vi "calculate_smooth_points.vi"(8 "error in (no error)":errorcluster, 11 "TrajectoryDL120126ArbitraryLine2D in":refnum<class "TrajectoryDL120126ArbitraryLine2D.lvclass">) -> (0 "error out":errorcluster, 2 "number of pixels":i32, 3 "TrajectoryDL120126ArbitraryLine2D out":refnum<class "TrajectoryDL120126ArbitraryLine2D.lvclass">)   [LabVIEW 2010, in "TrajectoryDL120126ArbitraryLine2D.lvclass"]
uses:
  TrajectoryDL120126ArbitraryLine2D.lvclass
  segment_cluster.ctl
  common/classes/SpaceVector/SpaceVector/SpaceVector.lvclass
  TrajectoryDL120126ArbitraryLine2D.lvclass/TrajectoryDL120126ArbitraryLine2D.ctl
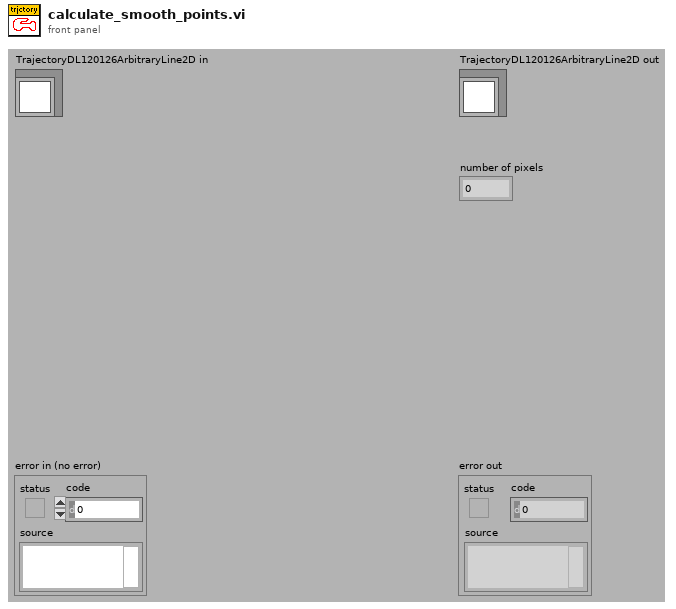
[diagram p1: front panel]
types:
  T1 = typedef "TrajectoryDL120126ArbitraryLine2D.lvclass/segment_cluster.ctl" = cluster{"points":refnum<class "SpaceVector.lvclass">[]}
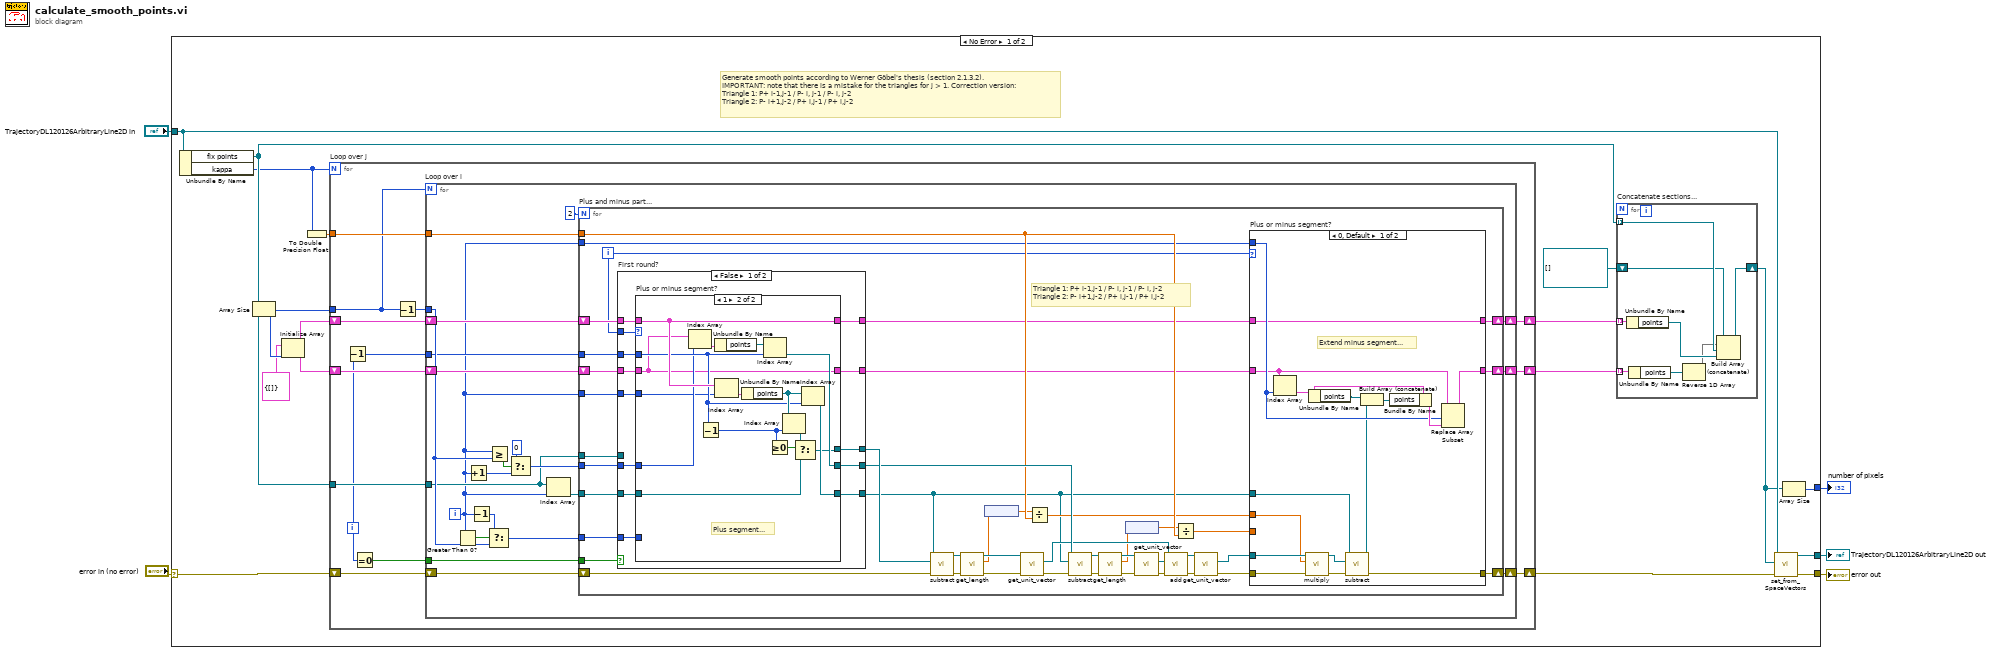
[diagram p0: block diagram]
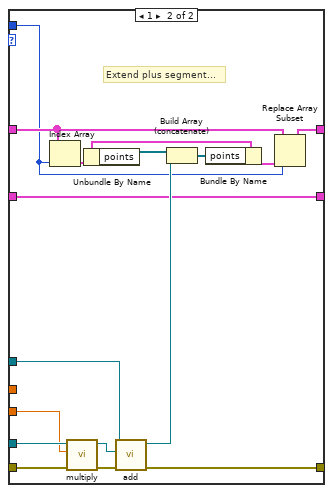
[diagram p2: hidden frame]
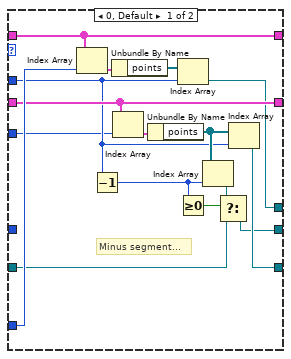
[diagram p3: hidden frame]
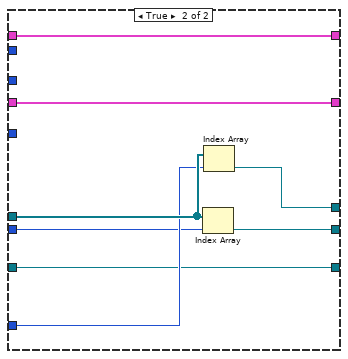
[diagram p4: hidden frame]
diagram:
  n1 = case shown="No Error" "error in (no error)" {
    selector: "error in (no error)" -> [w21 w192]
    tunnel: "TrajectoryDL120126ArbitraryLine2D in" -> [w11 w193]
    tunnel: [w9 w192] -> w3
    tunnel: [w10 w193] -> w2
    tunnel: [w6 _] -> w1
    frame No Error {
      # "Generate smooth points according to Werner Göbel's thesis (section 2.1.3.2). \nIMPORTANT: note that there is a mistake for the triangles for j > 1. Correction version:\nTriangle 1: P+ i-1,j-1 / P- i, j-1 / P- i, j-2\nTriangle 2: P- i+1,j-2 / P+ i,j-1 / P+ i,j-2"
      n2 = Unbundle By Name(w11) -> ("fix points"=w14:refnum<class "SpaceVector.lvclass">[], "kappa"=w13:i32)
      n3 = Array Size(array=w14) -> (size(s)=w18:i32)
      n4 = Initialize Array(T1 {"points"=[]} ("segment"), w18) -> (w16:T1[])
      n5 = To Double Precision Float(number=w13) -> (double precision float=w20:dbl)
      n6 = for "Loop over j" {
        N: w13 -> [_]
        tunnel: w14 -> [w40]
        shift-right: [w41] -> w12
        shift-left: w21 -> [w42]
        shift-right: [w38] -> w19
        shift-left: w16 -> [w39]
        shift-right: [w36] -> w8
        shift-left: w16 -> [w37]
        tunnel: w20 -> [w35]
        tunnel: w18 -> [w31]
        i -> [w33]
        n7 = Decrement(x=w33) -> (x-1=w34:i32)
        n8 = Equal To 0?(x=w33) -> (x = 0?=w32:bool)
        n9 = Decrement(x=w31) -> (x-1=w30:i32)
        n10 = for "Loop over i" {
          N: w31 -> [_]
          shift-right: [w61] -> w41
          shift-left: w42 -> [w63]
          tunnel: w40 -> [w46]
          shift-right: [w59] -> w38
          shift-left: w39 -> [w52]
          shift-right: [w60] -> w36
          shift-left: w37 -> [w50]
          tunnel: w35 -> [w62]
          tunnel: w30 -> [w49]
          tunnel: w34 -> [w47]
          tunnel: w32 -> [w45]
          i -> [w43]
          n11 = Greater Than 0?(x=w43) -> (x > 0?=w58:bool)
          n12 = Increment(x=w43) -> (x+1=w53:i32)
          n13 = Decrement(x=w43) -> (x-1=w57:i32)
          n14 = Select(t=w57, s=w58, f=w49) -> (s? t:f=w51:i32)
          n15 = Greater Or Equal?(x=w43, y=w49) -> (x >= y?=w56:bool)
          n16 = Select(t=0, s=w56, f=w53) -> (s? t:f=w55:i32)
          n17 = Index Array(array=w46, index=w43) -> (element=w48:refnum<class "SpaceVector.lvclass">)
          n18 = for "Plus and minus part..." {
            N: 2 -> [_]
            tunnel: w62 -> [w88]
            tunnel: w55 -> [w77]
            tunnel: w43 -> [w66]
            tunnel: w51 -> [w75]
            tunnel: w48 -> [w73]
            tunnel: w47 -> [w72]
            tunnel: w46 -> [w71]
            tunnel: w45 -> [w70]
            shift-right: [w78] -> w59
            shift-left: w52 -> [w76]
            shift-right: [w79] -> w60
            shift-left: w50 -> [w74]
            shift-right: [w80] -> w61
            shift-left: w63 -> [w104]
            tunnel: w43 -> [w65]
            i -> [w64]
            # "Triangle 1: P+ i-1,j-1 / P- i, j-1 / P- i, j-2\nTriangle 2: P- i+1,j-2 / P+ i,j-1 / P+ i,j-2"
            n19 = case "First round?" shown="False" w70 {
              tunnel: [w144 w187] -> w106
              tunnel: [w146 w188] -> w105
              tunnel: w77 -> [w142 w189]
              tunnel: w76 -> [w148 w185]
              tunnel: w75 -> [w151 w190]
              tunnel: w74 -> [w147 w184]
              tunnel: w73 -> [w150 w186]
              tunnel: w72 -> [w149 _]
              tunnel: w71 -> [_ w191]
              tunnel: [w145 w186] -> w69
              tunnel: [w140 w185] -> w68
              tunnel: [w139 w184] -> w67
              tunnel: w64 -> [w143 _]
              tunnel: w65 -> [w141 _]
              frame False {
                n20 = case "Plus or minus segment?" shown="1" w143 {
                  tunnel: w151 -> [w160 _]
                  tunnel: w150 -> [w159 w175]
                  tunnel: w149 -> [w157 w174]
                  tunnel: w148 -> [w156 w183]
                  tunnel: w147 -> [w158 w168]
                  tunnel: [w153 w173] -> w146
                  tunnel: [w155 w172] -> w145
                  tunnel: [w152 w171] -> w144
                  tunnel: w142 -> [_ w170]
                  tunnel: w141 -> [w154 w169]
                  tunnel: [w156 w183] -> w140
                  tunnel: [w158 w168] -> w139
                  frame 0, Default {
                    # "Minus segment..."
                    n21 = Index Array(array=w156, index=w160) -> (element=w167:T1)
                    n22 = Decrement(x=w157) -> (x-1=w163:i32)
                    n23 = Unbundle By Name(w167) -> ("points"=w166:refnum<class "SpaceVector.lvclass">[])
                    n24 = Index Array(array=w158, index=w154) -> (element=w165:T1)
                    n25 = Unbundle By Name(w165) -> ("points"=w164:refnum<class "SpaceVector.lvclass">[])
                    n26 = Index Array(array=w166, index=w157) -> (element=w152:refnum<class "SpaceVector.lvclass">)
                    n27 = Greater Or Equal To 0?(x=w163) -> (x >= 0?=w162:bool)
                    n28 = Index Array(array=w164, index=w163) -> (element=w161:refnum<class "SpaceVector.lvclass">)
                    n29 = Select(t=w161, s=w162, f=w159) -> (s? t:f=w153:refnum<class "SpaceVector.lvclass">)
                    n30 = Index Array(array=w164, index=w157) -> (element=w155:refnum<class "SpaceVector.lvclass">)
                  }
                  frame 1 {
                    # "Plus segment..."
                    n31 = Index Array(array=w168, index=w170) -> (element=w182:T1)
                    n32 = Decrement(x=w174) -> (x-1=w178:i32)
                    n33 = Unbundle By Name(w182) -> ("points"=w181:refnum<class "SpaceVector.lvclass">[])
                    n34 = Index Array(array=w183, index=w169) -> (element=w180:T1)
                    n35 = Unbundle By Name(w180) -> ("points"=w179:refnum<class "SpaceVector.lvclass">[])
                    n36 = Index Array(array=w181, index=w174) -> (element=w173:refnum<class "SpaceVector.lvclass">)
                    n37 = Greater Or Equal To 0?(x=w178) -> (x >= 0?=w177:bool)
                    n38 = Index Array(array=w179, index=w178) -> (element=w176:refnum<class "SpaceVector.lvclass">)
                    n39 = Select(t=w176, s=w177, f=w175) -> (s? t:f=w171:refnum<class "SpaceVector.lvclass">)
                    n40 = Index Array(array=w179, index=w174) -> (element=w172:refnum<class "SpaceVector.lvclass">)
                  }
                }
              }
              frame True {
                n41 = Index Array(array=w191, index=w189) -> (element=w188:refnum<class "SpaceVector.lvclass">)
                n42 = Index Array(array=w191, index=w190) -> (element=w187:refnum<class "SpaceVector.lvclass">)
              }
            }
            n43 = call "subtract.vi"("error in (no error)"=w104, "subtrahend"=w106, "SpaceVector in"=w69) -> ("error out"=w96:errorcluster, "SpaceVector out"=w97:refnum<class "SpaceVector.lvclass">)  [unwired: 7 in]
            n44 = call "get_length.vi"("error in (no error)"=w96, "SpaceVector in"=w97) -> ("error out"=w95:errorcluster, "length"=w89:dbl[unit], "SpaceVector out"=w94:refnum<class "SpaceVector.lvclass">)  [unwired: 7 in]
            n45 = node(w89) -> (w85:dbl)
            n46 = call "get_unit_vector.vi"("error in (no error)"=w95, "SpaceVector in"=w94) -> ("error out"=w103:errorcluster, "unit vector"=w101:refnum<class "SpaceVector.lvclass">)  [unwired: 7 in, 1 out]
            n47 = Divide(x=w85, y=w88) -> (x/y=w86:dbl)
            n48 = call "subtract.vi"("error in (no error)"=w103, "subtrahend"=w69, "SpaceVector in"=w105) -> ("error out"=w91:errorcluster, "SpaceVector out"=w93:refnum<class "SpaceVector.lvclass">)  [unwired: 7 in]
            n49 = call "get_length.vi"("error in (no error)"=w91, "SpaceVector in"=w93) -> ("error out"=w90:errorcluster, "length"=w84:dbl[unit], "SpaceVector out"=w92:refnum<class "SpaceVector.lvclass">)  [unwired: 7 in]
            n50 = node(w84) -> (w83:dbl)
            n51 = call "get_unit_vector.vi"("error in (no error)"=w90, "SpaceVector in"=w92) -> ("error out"=w100:errorcluster, "unit vector"=w102:refnum<class "SpaceVector.lvclass">)  [unwired: 7 in, 1 out]
            n52 = call "add.vi"("error in (no error)"=w100, "vector to be added"=w102, "SpaceVector in"=w101) -> ("error out"=w98:errorcluster, "SpaceVector out"=w99:refnum<class "SpaceVector.lvclass">)  [unwired: 7 in]
            n53 = Divide(x=w83, y=w88) -> (x/y=w81:dbl)
            n54 = call "get_unit_vector.vi"("error in (no error)"=w98, "SpaceVector in"=w99) -> ("error out"=w87:errorcluster, "unit vector"=w82:refnum<class "SpaceVector.lvclass">)  [unwired: 7 in, 1 out]
            n55 = case "Plus or minus segment?" shown="0, Default" w64 {
              tunnel: w87 -> [w114 w123]
              tunnel: w86 -> [w110 _]
              tunnel: w82 -> [w111 w138]
              tunnel: w81 -> [_ w137]
              tunnel: [w112 w134] -> w80
              tunnel: [w118 w124] -> w79
              tunnel: [w116 w131] -> w78
              tunnel: w69 -> [w109 w127]
              tunnel: w68 -> [w116 w126]
              tunnel: w67 -> [w117 w124]
              tunnel: w66 -> [w119 w125]
              frame 0, Default {
                # "Extend minus segment..."
                n56 = Index Array(array=w117, index=w119) -> (element=w122:T1)
                n57 = call "multiply.vi"("error in (no error)"=w114, "factor"=w110, "SpaceVector in"=w111) -> ("error out"=w113:errorcluster, "SpaceVector out"=w115:refnum<class "SpaceVector.lvclass">)  [unwired: 7 in]
                n58 = Unbundle By Name(w122) -> ("points"=w107:refnum<class "SpaceVector.lvclass">[])
                n59 = call "subtract.vi"("error in (no error)"=w113, "subtrahend"=w115, "SpaceVector in"=w109) -> ("error out"=w112:errorcluster, "SpaceVector out"=w108:refnum<class "SpaceVector.lvclass">)  [unwired: 7 in]
                n60 = Build Array (concatenate)(w107, w108) -> (w121:refnum<class "SpaceVector.lvclass">[])
                n61 = Bundle By Name(cluster=w122, "points"=w121) -> (w120:T1)
                n62 = Replace Array Subset(array=w117, new element=w120, index=w119) -> (w118:T1[])
              }
              frame 1 {
                # "Extend plus segment..."
                n63 = Index Array(array=w126, index=w125) -> (element=w130:T1)
                n64 = call "multiply.vi"("error in (no error)"=w123, "factor"=w137, "SpaceVector in"=w138) -> ("error out"=w135:errorcluster, "SpaceVector out"=w136:refnum<class "SpaceVector.lvclass">)  [unwired: 7 in]
                n65 = Unbundle By Name(w130) -> ("points"=w129:refnum<class "SpaceVector.lvclass">[])
                n66 = call "add.vi"("error in (no error)"=w135, "vector to be added"=w136, "SpaceVector in"=w127) -> ("error out"=w134:errorcluster, "SpaceVector out"=w128:refnum<class "SpaceVector.lvclass">)  [unwired: 7 in]
                n67 = Build Array (concatenate)(w129, w128) -> (w132:refnum<class "SpaceVector.lvclass">[])
                n68 = Bundle By Name(cluster=w130, "points"=w132) -> (w133:T1)
                n69 = Replace Array Subset(array=w126, new element=w133, index=w125) -> (w131:T1[])
              }
            }
          }
        }
      }
      n70 = for "Concatenate sections..." {
        tunnel: w14 -> [w27] mode=indexing
        shift-right: [w24] -> w7
        shift-left: refnum<class "SpaceVector.lvclass">[] [] -> [w25]
        tunnel: w19 -> [w29] mode=indexing
        tunnel: w8 -> [w28] mode=indexing
        n71 = Unbundle By Name(w29) -> ("points"=w26:refnum<class "SpaceVector.lvclass">[])
        n72 = Unbundle By Name(w28) -> ("points"=w23:refnum<class "SpaceVector.lvclass">[])
        n73 = Reverse 1D Array(array=w23) -> (reversed array=w22:refnum<class "SpaceVector.lvclass">[])
        n74 = Build Array (concatenate)(w25, w22, w27, w26) -> (w24:refnum<class "SpaceVector.lvclass">[])
      }
      n75 = call-dynamic "set_from_SpaceVectors.vi"("error in (no error)"=w12, "voxels"=w7, "TrajectoryDL091126GenericVoxel in"=w11) -> ("error out"=w9:errorcluster, "TrajectoryDL091126GenericVoxel out"=w10:refnum<class "TrajectoryDL120126ArbitraryLine2D.lvclass">)  [unwired: 7 in]
      n76 = Array Size(array=w7) -> (size(s)=w6:i32)
    }
    frame Error {
    }
  }
  "error out" <- w3
  "TrajectoryDL120126ArbitraryLine2D out" <- w2
  "number of pixels" <- w1
